vi "strom-akku.vi"(11 "Dynamic Data":dynamicdata(waveform)) -> (3 "Filtered Signal":dynamicdata(waveform))   [LabVIEW 2018]
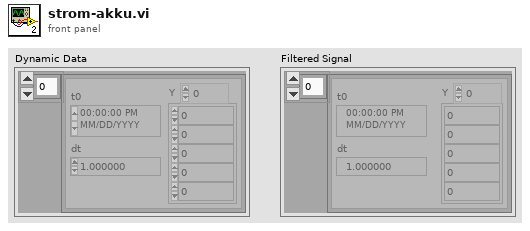
[diagram p1: front panel]
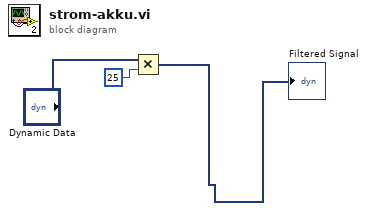
[diagram p0: block diagram]
diagram:
  n1 = Multiply(x="Dynamic Data", y=25) -> (x*y=→"Filtered Signal":dynamicdata)
